vi "Identify Request.vi"(8 "error in (no error)":errorcluster, 11 "Request in":refnum<class "Request.lvclass">) -> (0 "error out":errorcluster, 1 "params":variant, 2 "method":string, 3 "Request out":refnum<class "Request.lvclass">, 4 "id value":string)   [LabVIEW 2020, in "RPC.lvlib"]
uses:
  RPC.lvlib
  External/JSON-RPC/Classes/Request/Request.lvclass
  External/JSON-RPC/Classes/Request/Request.lvclass/Request.ctl
  TypeDefs/ServerMethods.ctl
  External/JSON-RPC/Classes/Request/request.Read method.vi
  External/JSON-RPC/Classes/Request/request.Read params.vi
  External/JSON-RPC/Classes/Request/request.Has ID.vi
  External/JSON-RPC/Classes/params/params.To JSON Tree.vi
  External/JSON-RPC/Classes/Request/request.Read id value.vi
  External/JSON-RPC/Classes/id/id.Read value.vi
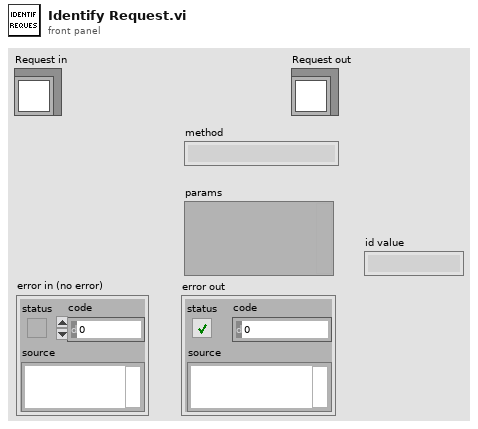
[diagram p1: front panel]
types:
  T1 = typedef "RPC.lvlib/ServerMethods.ctl" = string
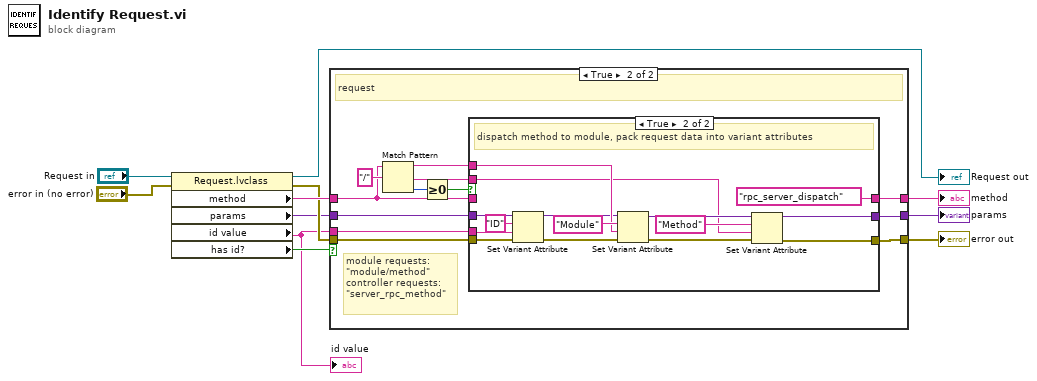
[diagram p0: block diagram]
diagram:
  n1 = property class="Request.lvclass"(reference="Request in", error in="error in (no error)") -> (reference out=→"Request out":refnum<class "Request.lvclass">, error out=w8:errorcluster, "method"=w10:string, "params"=w7:variant, "id value"=w2:string, "has id?"=w3:bool)
  "id value" <- w2
  n2 = case shown="True" w3 {
    tunnel: w10 -> [w12 w23]
    tunnel: w8 -> [w13 w16]
    tunnel: w7 -> [w14 w17]
    tunnel: [w14 w20] -> w6
    tunnel: [w13 w21] -> w5
    tunnel: [w12 w19] -> w4
    tunnel: w2 -> [_ w15]
    frame False {
      # "notification"
    }
    frame True {
      # "module requests:\n\"module/method\"\ncontroller requests:\n\"server_rpc_method\""
      # "request"
      n3 = Match Pattern(string=w23, regular expression="/") -> (before substring=w22:string, after substring=w24:string, offset past match=w25:i32)  [unwired: 1 in, 1 out]
      n4 = Greater Or Equal To 0?(x=w25) -> (x >= 0?=w18:bool)
      n5 = case shown="True" w18 {
        tunnel: w24 -> [_ w37]
        tunnel: w23 -> [w29 _]
        tunnel: w22 -> [_ w40]
        tunnel: [w27 w39] -> w21
        tunnel: [w28 w38] -> w20
        tunnel: [w29 T1 "rpc_server_dispatch" ("method")] -> w19
        tunnel: w17 -> [w28 w33]
        tunnel: w16 -> [w27 w32]
        tunnel: w15 -> [_ w31]
        frame False {
          # "controller method"
        }
        frame True {
          # "dispatch method to module, pack request data into variant attributes"
          n6 = Set Variant Attribute(Variant=w33, name="ID", value=w31, error in=w32) -> (Variant out=w35:variant, error out=w34:errorcluster)  [unwired: 1 out]
          n7 = Set Variant Attribute(Variant=w35, name="Module", value=w40, error in=w34) -> (Variant out=w41:variant, error out=w44:errorcluster)  [unwired: 1 out]
          n8 = Set Variant Attribute(Variant=w41, name="Method", value=w37, error in=w44) -> (Variant out=w38:variant, error out=w39:errorcluster)  [unwired: 1 out]
        }
      }
    }
  }
  "params" <- w6
  "error out" <- w5
  "method" <- w4
